vi "Simple Class-Based Logging.vi"() -> ()   [LabVIEW 2018]
uses:
  src/api/Log Levels.ctl
  ff44e4a9-c346-414c-ae2a-efcf3ff82913.vi
  src/api/GLog.lvlib
  src/api/logger_class/Logger.lvclass
panel:
  in  "error in (no error)":errorcluster
  out "error out":errorcluster
  in  "total iterations":i32=30
  # "Locals"
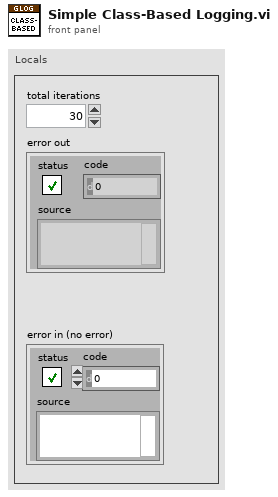
[diagram p1: front panel]
types:
  T1 = typedef "GLog.lvlib/Log Levels.ctl" = enum16{"Trace", "Debug", "Info", "Warning", "Error", "Critical"}
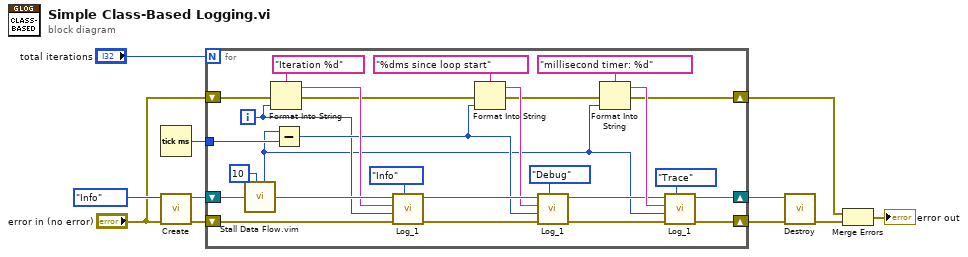
[diagram p0: block diagram]
diagram:
  n1 = Tick Count (ms)() -> (millisecond timer value=w11:u32)
  n2 = call "Create.vi"("error in (no error)"="error in (no error)", "minimum log level (Info)"=Log_Levels."Info" ("minimum log level")) -> ("error out"=w5:errorcluster, "logger"=w6:refnum<class "Logger.lvclass">)  [unwired: 8 in]
  n3 = for {
    N: "total iterations" -> [_]
    shift-right: [w22] -> w9
    shift-left: w6 -> [w33]
    tunnel: w11 -> [w36]
    shift-right: [w16] -> w8
    shift-left: w5 -> [w19]
    shift-right: [w12] -> w1
    shift-left: "error in (no error)" -> [w15]
    i -> [w27]
    n4 = call "Stall Data Flow.vim"("value in"=w33, "milliseconds to wait"=u32 10 ("loop iteration delay [ms]")) -> ("millisecond timer value"=w21:u32, "value out"=w35:refnum<class "Logger.lvclass">)
    n5 = Format Into String(format string="Iteration %d" ("message"), error in=w15, w27) -> (resulting string=w31:string, error out=w14:errorcluster)  [unwired: 1 in]
    n6 = Subtract(x=w21, y=w36) -> (x-y=w28:u32)
    n7 = call "Log_1.vi"("log level"=Log_Levels."Info", "error in"=w19, "data (null)"=w27, "message"=w31, "logger in"=w35) -> ("error out"=w18:errorcluster, "logger out"=w38:refnum<class "Logger.lvclass">)  [unwired: 5 in]
    n8 = Format Into String(format string="%dms since loop start" ("message"), error in=w14, w28) -> (resulting string=w29:string, error out=w13:errorcluster)  [unwired: 1 in]
    n9 = call "Log_1.vi"("log level"=Log_Levels."Debug", "error in"=w18, "data (null)"=w28, "message"=w29, "logger in"=w38) -> ("error out"=w17:errorcluster, "logger out"=w23:refnum<class "Logger.lvclass">)  [unwired: 5 in]
    n10 = Format Into String(format string="millisecond timer: %d" ("message"), error in=w13, w21) -> (resulting string=w26:string, error out=w12:errorcluster)  [unwired: 1 in]
    n11 = call "Log_1.vi"("log level"=Log_Levels."Trace", "error in"=w17, "data (null)"=w21, "message"=w26, "logger in"=w23) -> ("error out"=w16:errorcluster, "logger out"=w22:refnum<class "Logger.lvclass">)  [unwired: 5 in]
  }
  n12 = call "Destroy.vi"("error in (no error)"=w8, "logger in"=w9) -> ("error out"=w7:errorcluster)  [unwired: 8 in, 1 out]
  n13 = Merge Errors(w1, w7) -> (→"error out":errorcluster)
